vi "mxwScript_API_XMLTemplateName_DropBesideNodeTerminal.vi"(5 "direction":T1, 7 "distance":i32 min=0, 8 "error in (no error)":errorcluster, 9 "nodeTerminalID":string, 10 "templateTerminalPath":string, 11 "absolutePath":string) -> (0 "error out":errorcluster, 3 "encoded absolutePath":string)   [LabVIEW 2020]
doc: "Add diagram to drop this template into to the template name."
uses:
  codeGenAPISupport.llb/cgAPI_mxwScript_DrpTmplt_SimpleDirection.ctl
  codeGenAPISupport.llb/cgAPI_mxwScript_DrpTmplt_TargetRefType.ctl
  codeGenAPISupport.llb/cgAPI_mxwScript_DrpTmplt_TemplateRefType.ctl
  codeGenAPISupport.llb/cgAPI_mxwScript_DrpTmplt_TerminalData.ctl
  codeGenAPISupport.llb/cgAPI_mxwScript_DrpTmplt_ReferencePosition.ctl
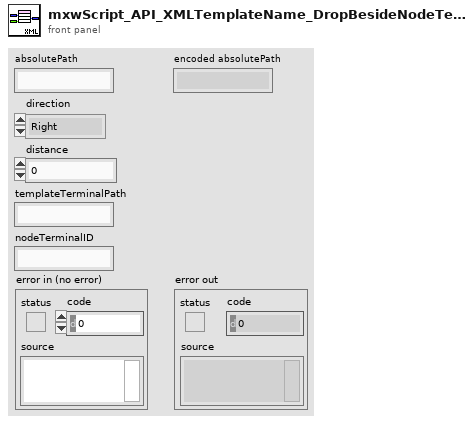
[diagram p1: front panel]
types:
  T1 = typedef "cgAPI_mxwScript_DrpTmplt_SimpleDirection.ctl" = enum16{"Right", "Left", "Below", "Above"}
  T2 = typedef "cgAPI_mxwScript_DrpTmplt_TerminalData.ctl" = cluster{"name":string, "termIsTag":bool, "referencePosition":T3}
  T3 = typedef "cgAPI_mxwScript_DrpTmplt_ReferencePosition.ctl" = enum16{"TopLeft", "Top", "TopRight", "Left", "Middle", "Right", "BottomLeft", "Bottom", "BottomRight"}
  T4 = typedef "cgAPI_mxwScript_DrpTmplt_TemplateRefType.ctl" = enum16{"InputAverage", "Absolute", "Terminal"}
  T5 = typedef "cgAPI_mxwScript_DrpTmplt_TargetRefType.ctl" = enum16{"RelativeToTemplate", "RelativeToTerminal", "AbsoluteOnRoot", "AbsoluteOnTarget", "RelativeToExistOnRoot"}
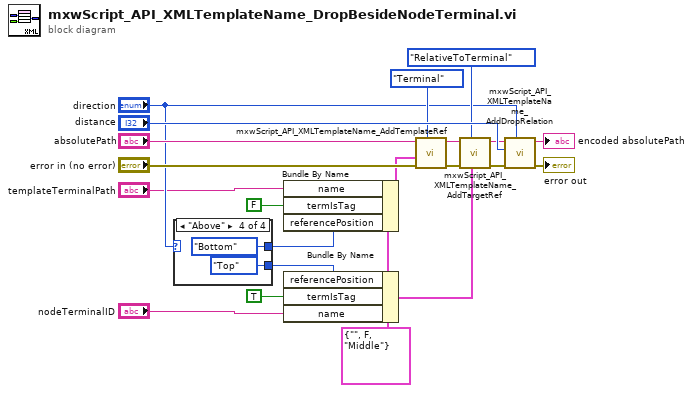
[diagram p0: block diagram]
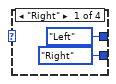
[diagram p2: hidden frame]
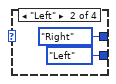
[diagram p3: hidden frame]
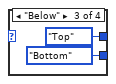
[diagram p4: hidden frame]
diagram:
  w9 = T2 {"name"="", "termIsTag"=FALSE, "referencePosition"=enum."Middle"} ("terminalData")
  n1 = case shown="\"Above\"" "direction" {
    tunnel: [cgAPI_mxwScript_DrpTmplt_ReferencePosition."Left" ("referencePosition") cgAPI_mxwScript_DrpTmplt_ReferencePosition."Right" ("referencePosition") cgAPI_mxwScript_DrpTmplt_ReferencePosition."Top" ("referencePosition") cgAPI_mxwScript_DrpTmplt_ReferencePosition."Bottom" ("referencePosition")] -> w7
    tunnel: [cgAPI_mxwScript_DrpTmplt_ReferencePosition."Right" ("referencePosition") cgAPI_mxwScript_DrpTmplt_ReferencePosition."Left" ("referencePosition") cgAPI_mxwScript_DrpTmplt_ReferencePosition."Bottom" ("referencePosition") cgAPI_mxwScript_DrpTmplt_ReferencePosition."Top" ("referencePosition")] -> w6
    frame "Right" {
    }
    frame "Left" {
    }
    frame "Below" {
    }
    frame "Above" {
    }
  }
  n2 = Bundle By Name(cluster=w9, "name"="templateTerminalPath", "termIsTag"=FALSE, "referencePosition"=w7) -> (w10:T2)
  n3 = Bundle By Name(cluster=w9, "referencePosition"=w6, "termIsTag"=TRUE, "name"="nodeTerminalID") -> (w8:T2)
  n4 = call "mxwScript_API_XMLTemplateName_AddTemplateRef.vi"("templateRefType"=cgAPI_mxwScript_DrpTmplt_TemplateRefType."Terminal", "error in (no error)"="error in (no error)", "terminalData"=w10, "absolutePath"="absolutePath") -> ("error out"=w15:errorcluster, "encoded absolutePath"=w14:string)  [unwired: 1 in, 5 out]
  n5 = call "mxwScript_API_XMLTemplateName_AddTargetRef.vi"("terminalData"=w8, "targetRefType"=cgAPI_mxwScript_DrpTmplt_TargetRefType."RelativeToTerminal", "error in (no error)"=w15, "absolutePath"=w14) -> ("error out"=w18:errorcluster, "encoded absolutePath"=w17:string)  [unwired: 3 in, 3 out]
  n6 = call "mxwScript_API_XMLTemplateName_AddDropRelation.vi"("direction"="direction", "error in (no error)"=w18, "distance"="distance", "absolutePath"=w17) -> ("error out"=→"error out":errorcluster, "encoded absolutePath"=→"encoded absolutePath":string)  [unwired: 1 in, 5 out]
